vi "convert timespec to nanoseconds.vi"(11 "timespec":cluster{"sec":u64, "nsec":u64}) -> (3 "nanoseconds":i64)   [LabVIEW 2013, in "Linux RT Utilities.lvlib"]
uses:
  Linux RT Utilities.lvlib
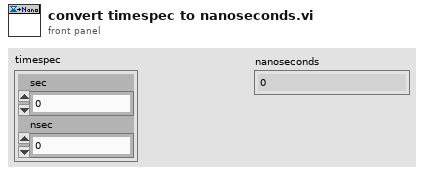
[diagram p1: front panel]
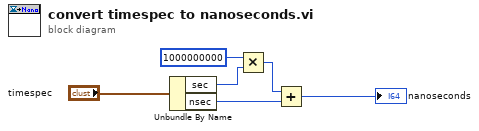
[diagram p0: block diagram]
diagram:
  n1 = Unbundle By Name("timespec") -> ("sec"=w4:u64, "nsec"=w2:u64)
  n2 = Multiply(x=i64 1000000000, y=w4) -> (x*y=w1:u64)
  n3 = Add(x=w1, y=w2) -> (x+y=→"nanoseconds":u64)
